vi "Gyro Zero Button.vi"(8 "error in":errorcluster, 11 "Boolean":bool) -> ()   [LabVIEW 2017]
uses:
  FRC3026/PowerUp/navx-mxp/labview/navX Library v2/navX Library v2.lvlib
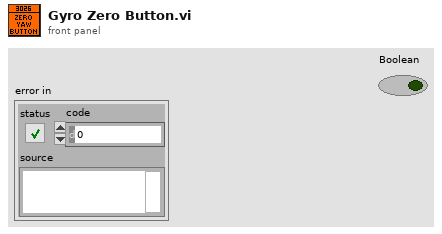
[diagram p1: front panel]
types:
  T1 = typedef "navX Library v2.lvlib/Z900_navX_DeviceTypeDef.ctl" = cluster{"Interface":cluster{"Protocol":T2, "Update Rate (4Hz-100Hz)":u8, "navX Open TypeDef":variant}, "Notify Packet":refnum<notifier>, "Loop VI Refnum":refnum<vi>, "Ready to Close Occurrence Refnum":refnum<k4>}
  T2 = typedef "navX Library v2.lvlib/Z900_navX_ProtocolTypeDef.ctl" = enum16{"SERIAL", "I2C", "SPI"}
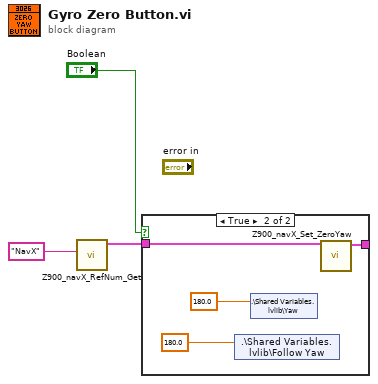
[diagram p0: block diagram]
diagram:
  n1 = call "Z900_navX_RefNum_Get.vi"("refnum name"="NavX") -> ("navX Device"=w1:T1)  [unwired: 9 in, 1 out]
  n2 = case shown="True" "Boolean" {
    tunnel: [w4 w6] -> _
    tunnel: w1 -> [w4 w5]
    frame False {
    }
    frame True {
      n3 = shared-variable ".\\Shared Variables.lvlib\\Follow Yaw"(180.0 ("Follow Yaw")) -> ()  [unwired: 1 in, 1 out]
      n4 = shared-variable ".\\Shared Variables.lvlib\\Yaw"(180.0 ("Yaw")) -> ()  [unwired: 1 in, 1 out]
      n5 = call "Z900_navX_Set_ZeroYaw.vi"("navX Device"=w5) -> ("navX Device"=w6:T1)  [unwired: 9 in, 1 out]
    }
  }
